vi "TEST_DataQ 1.vi"() -> ()   [LabVIEW 2024]
panel:
  in  "Fill":bool
  out "Message":string[](array[string])
  in  "stop":bool
  out "ChB Ohms":dbl=-0.0749980268396874 format="%.1f"
  out "ChA Ohms":dbl=-0.05868109013049169 format="%.1f"
  in  "State Msg":enum16{"INIT", "IDLE", "STOP", "FILL", "DRAIN"}(ring)
  out "DataQ":bool=TRUE
  in  "Drain":bool
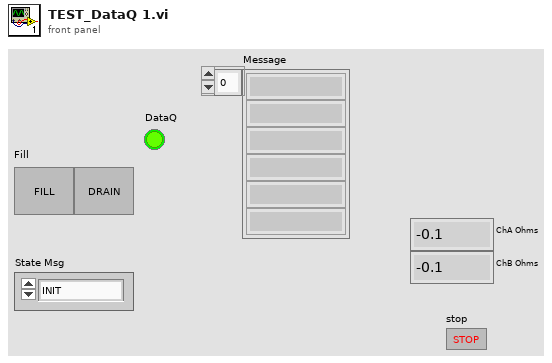
[diagram p1: front panel]
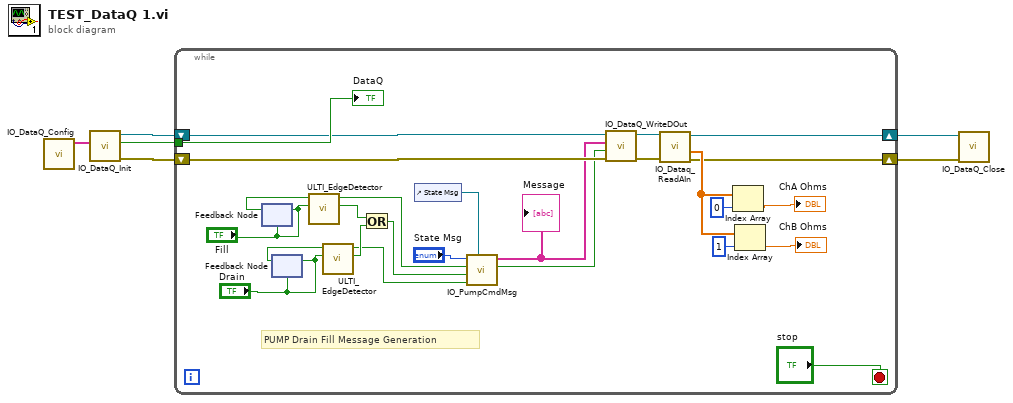
[diagram p0: block diagram]
diagram:
  n1 = call "IO_DataQ_Config.vi"() -> ("Init Message"=w6:string[])  [unwired: 11 in]
  n2 = call "IO_DataQ_Init.vi"("Command\nList"=w6) -> ("error out"=w2:errorcluster, "Connected?"=w3:bool, "VISA resource name out"=w1:refnum<visa-resource-name>)  [unwired: 8 in]
  n3 = while {
    tunnel: w3 -> [w14]
    shift-right: [w18] -> w5
    shift-left: w2 -> [w13]
    shift-right: [w17] -> w4
    shift-left: w1 -> [w12]
    stop <- "stop" stop-if-true
    # "PUMP Drain Fill Message Generation"
    n4 = feedback #1("Fill") -> (w31:bool)
    n5 = feedback-in #1("Fill") -> ()
    n6 = feedback #2("Drain") -> (w32:bool)
    n7 = feedback-in #2("Drain") -> ()
    n8 = call "ULTI_EdgeDetector.vi"("IN (N)"="Fill", "IN (N+2)"=w31) -> ("Neg Edge"=w29:bool, "Pos Edge"=w28:bool)  [unwired: 8 in]
    n9 = call "ULTI_EdgeDetector.vi"("IN (N)"="Drain", "IN (N+2)"=w32) -> ("Neg Edge"=w27:bool, "Pos Edge"=w26:bool)  [unwired: 8 in]
    n10 = Or(x=w29, y=w27) -> (x .or. y?=w30:bool)
    n11 = control-ref of="State Msg"() -> (w8:refnum<vi>)
    n12 = call "IO_PumpCmdMsg.vi"("State Ref"=w8, "Drain Signal"=w26, "Stop Signal"=w30, "FIll Signal"=w28, "State\n in"="State Msg") -> ("Msg Active"=w10:bool, "Message"=w11:string[])  [unwired: 5 in]
    "Message" <- w11
    n13 = call "IO_DataQ_WriteDOut.vi"("error in (no error)"=w13, "Msg Active"=w10, "Message"=w11, "VISA Refnum in"=w12) -> ("error out"=w20:errorcluster, "VISA Refnum out"=w19:refnum<visa-resource-name>)  [unwired: 5 in, 1 out]
    n14 = call "IO_Dataq_ReadAIn.vi"("error in (no error)"=w20, "VISA Refnum in"=w19) -> ("error out"=w18:errorcluster, "Outputs"=w21:dbl[], "VISA Refnum out"=w17:refnum<visa-resource-name>)  [unwired: 5 in, 2 out]
    n15 = Index Array(array=w21, index=0) -> (element=→"ChA Ohms":dbl)
    n16 = Index Array(array=w21, index=1) -> (element=→"ChB Ohms":dbl)
    "DataQ" <- w14
  }
  n17 = call "IO_DataQ_Close.vi"("error in"=w5, "VISA resource name"=w4) -> ()  [unwired: 9 in, 1 out]
